vi "Get.vi"(8 "error in (no error)":errorcluster, 10 "Command":string, 11 "Handle in":i32) -> (0 "error out":errorcluster, 2 "Returned String":string, 3 "Handle out":i32)   [LabVIEW 2013, in "Thorlabs_MC2000B.lvlib"]
uses:
  <instrlib>/Thorlabs_MC2000B/Thorlabs_MC2000B.lvlib
  <instrlib>/Thorlabs_MC2000B/Library/MC2000CommandLibWin64.dll
  <instrlib>/Thorlabs_MC2000B/Library/MC2000CommandLibWin32.dll
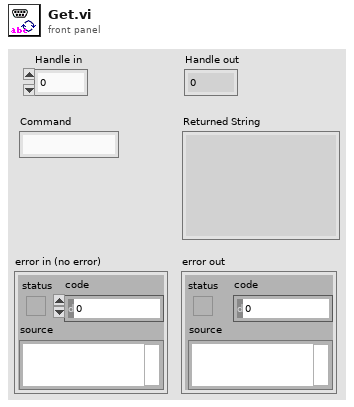
[diagram p1: front panel]
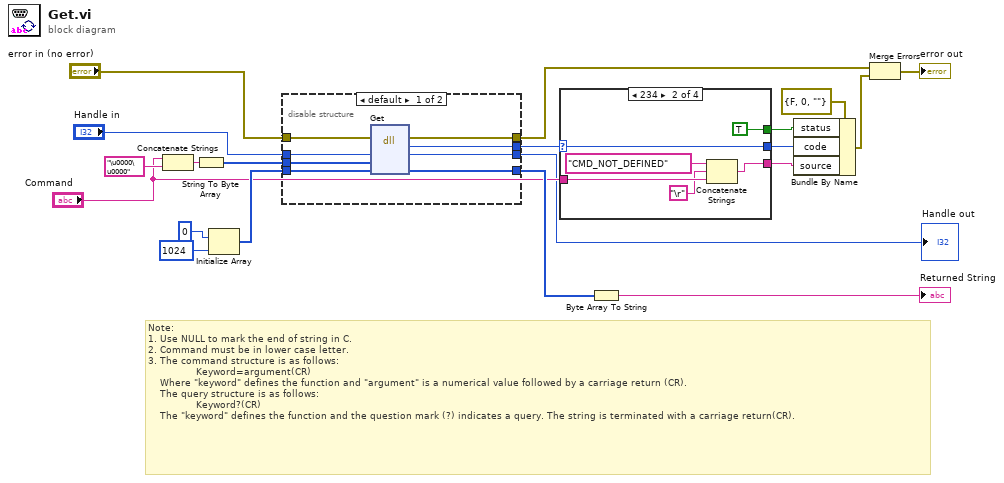
[diagram p0: block diagram]
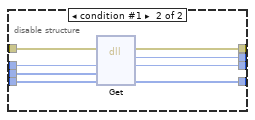
[diagram p2: hidden frame]
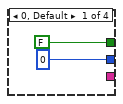
[diagram p3: hidden frame]
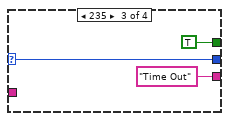
[diagram p4: hidden frame]
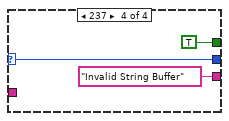
[diagram p5: hidden frame]
diagram:
  # "Note:\n1. Use NULL to mark the end of string in C.\n2. Command must be in lower case letter.\n3. The command structure is as follows:\n                Keyword=argument(CR)\n    Where \"keyword\" defines the function and \"argument\" is a numerical value followed by a carriage return (CR).\n    The query structure is as follows:\n                Keyword?(CR)\n    The \"keyword\" defines the function and the question mark (?) indicates a query. The string is terminated with a carriage return(CR)."
  n1 = Concatenate Strings("Command", "\u0000\u0000") -> (w19:string)
  n2 = String To Byte Array(string=w19) -> (unsigned byte array=w18:u8[])
  n3 = Initialize Array(u8 0, 1024 ("dimension size")) -> (w12:u8[])
  n4 = disable-structure shown="default" {
    disable-tunnel: w18 -> [w28 w36]
    disable-tunnel: [w27 w35] -> w17
    disable-tunnel: [w26 w34] -> w16
    disable-tunnel: w12 -> [w25 w33]
    disable-tunnel: "error in (no error)" -> [w24 w32]
    disable-tunnel: [w23 w31] -> w6
    disable-tunnel: "Handle in" -> [w22 w30]
    disable-tunnel: [w21 w29] -> w1
    frame condition #0 (active) {
      n5 = dll-call lib="C:/Program Files (x86)/National Instruments/LabVIEW 2013/instr.lib/Thorlabs_MC2000B/Library/MC2000CommandLibWin32.dll" fn="Get"(error in=w24, "hdl"=w22, "Input Command"=w28, "Returned String"=w25) -> (error out=w23:errorcluster, "return type"=w27:i32, "hdl"=w21:i32, "Returned String"=w26:u8[])  [unwired: 3 in, 1 out]
    }
    frame condition #1 {
      n6 = dll-call lib="D:/Program Files/National Instruments/LabVIEW 2011/instr.lib/Thorlabs_MC2000B/Library/MC2000CommandLibWin64.dll" fn="Get"(error in=w32, "hdl"=w30, "Input Command"=w36, "Returned String"=w33) -> (error out=w31:errorcluster, "return type"=w35:i32, "hdl"=w29:i32, "Returned String"=w34:u8[])  [unwired: 3 in, 1 out]
    }
  }
  "Handle out" <- w1
  n7 = case shown="234" w17 {
    selector: w17 -> [_ w43 w45 w48]
    tunnel: [_ w39 "Time Out" "Invalid String Buffer"] -> w7
    tunnel: [FALSE TRUE TRUE TRUE] -> w9
    tunnel: [0 w43 w45 w48] -> w8
    tunnel: "Command" -> [_ w41 _ _]
    frame 0, Default {
    }
    frame 234 {
      n8 = Concatenate Strings("CMD_NOT_DEFINED", "\r", w41) -> (w39:string)
    }
    frame 235 {
    }
    frame 237 {
    }
  }
  n9 = Byte Array To String(unsigned byte array=w16) -> (string=→"Returned String":string)
  n10 = Bundle By Name(cluster=errorcluster {"status"=FALSE, "code"=0, "source"=""} ("error out"), "status"=w9, "code"=w8, "source"=w7) -> (w5:errorcluster)
  n11 = Merge Errors(w6, w5) -> (→"error out":errorcluster)
